vi "Get Help.vi"(0 "Display State In":T1, 9 "Container State":T3, 11 "error in (no error)":errorcluster) -> (4 "Display State Out":T1, 6 "Help":string, 15 "error out":errorcluster)   [LabVIEW 2021, in "myRIO Channel Name.xctl"]
uses:
  <vilib>/myRIO/Common/Express VI Framework/xctls/myRIO Channel Name/myRIO Channel Name.xctl
  <vilib>/_xctls/Container State.ctl
  <vilib>/myRIO/Common/Express VI Framework/xctls/myRIO Channel Name/State.ctl
  <vilib>/myRIO/Common/Express VI Framework/typedefs/Data Validate Ref.ctl
  <vilib>/_xctls/XControlSupport.lvlib
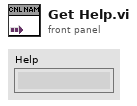
[diagram p1: front panel]
types:
  T1 = typedef "myRIO Channel Name.xctl/State.ctl" = cluster{"Channel Names":string[], "Data Valid":T2, "Current Channel":string}
  T2 = typedef "Data Validate Ref.ctl" = refnum<user-event>
  T3 = typedef "XControlSupport.lvlib/Container State.ctl" = cluster{"Indicator?":bool, "Run Mode?":bool, " Refnum":refnum<vi>}
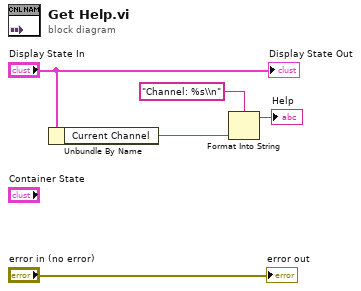
[diagram p0: block diagram]
diagram:
  n1 = Unbundle By Name("Display State In") -> ("Current Channel"=w2:string)
  n2 = Format Into String(format string="Channel: %s\\n", w2) -> (resulting string=→"Help":string)  [unwired: 2 in, 1 out]
  "Display State Out" <- "Display State In"
  "error out" <- "error in (no error)"
